vi "EIC_DIRC_DAQ_labview - kiethley.vi"() -> ()   [LabVIEW 2024]
uses:
  <instrlib>/Keithley 6517/Keithley 6517.lvlib
  O:/DSG/Tyler/EIC/DIRC/daq/automated/Thorlabs.MotionControl.Controls.dll
  Thorlabs.MotionControl.Controls.dll
  O:/DSG/Tyler/EIC/DIRC/daq/automated/Thorlabs.MotionControl.IntegratedStepperMotorsCLI.dll
  Thorlabs.MotionControl.IntegratedStepperMotorsCLI.dll
  O:/DSG/Tyler/EIC/DIRC/daq/automated/Thorlabs.MotionControl.DeviceManagerCLI.dll
  Thorlabs.MotionControl.DeviceManagerCLI.dll
panel:
  out "pdx_pos":dbl
  out "GetPositionCounter":i32
  out "pdy_dev":refnum<k24>
  out "pdx_dev":refnum<k24>
  in  "auto-align":bool
  out "meter-ref":string
  out "pd_rot_error":errorcluster
  out "brewster_rot_error":errorcluster
  in  "PD X":refnum<k24>(container)
  out "pd_rot_ref":refnum<k24>
  out "brewster_rot_ref":refnum<k24>
  in  "PD Angle":refnum<k24>(container)
  in  "Brewster":refnum<k24>(container)
  out "bary_error":errorcluster
  out "bary_ref":refnum<k24>
  out "barx_error":errorcluster
  out "barx_ref":refnum<k24>
  out "pdy_error":errorcluster
  out "pdy_ref":refnum<k24>
  out "pdx_error":errorcluster
  out "pdx_ref":refnum<k24>
  out "serial-numbers":string[](array[string])=["45000001", "45000002", "45000003", "45000004"]
  out "sim-instance":refnum<k24>
  in  "BAR Y":refnum<k24>(container)
  in  "BAR X":refnum<k24>(container)
  in  "PD Y":refnum<k24>(container)
  in  "dev-mode":bool
  out "start-msg":string
  in  "nSamples":dbl=50.0 caption="# Samples"
  in  "bar-note":bool
  out "sensor-stat":bool caption="Log Status"
  out "fout-stat":bool caption="Log Status"
  out "last-save":string caption="Last Save:"
  in  "save-data":bool
  out "Current Time:":string
  out "file-error":errorcluster
  out "log-path":path caption="Data will be saved at:"
  out "meter-error":errorcluster
  out "pd1_v":dbl caption="PD 1" format="%#.4g"
  out "pd2_v":dbl caption="PD 2" format="%#.4g"
  out "pd3_v":dbl caption="PD 3" format="%#.4g"
  out "pd-plt":cluster{"[0]":dbl, "[1]":dbl, "[2]":dbl}(graph) caption="Measurement History"
  in  "stop":bool
  # "PRESS STOP BEFORE \nCLOSING WINDOW"
  # "A"
  # "A"
  # "A"
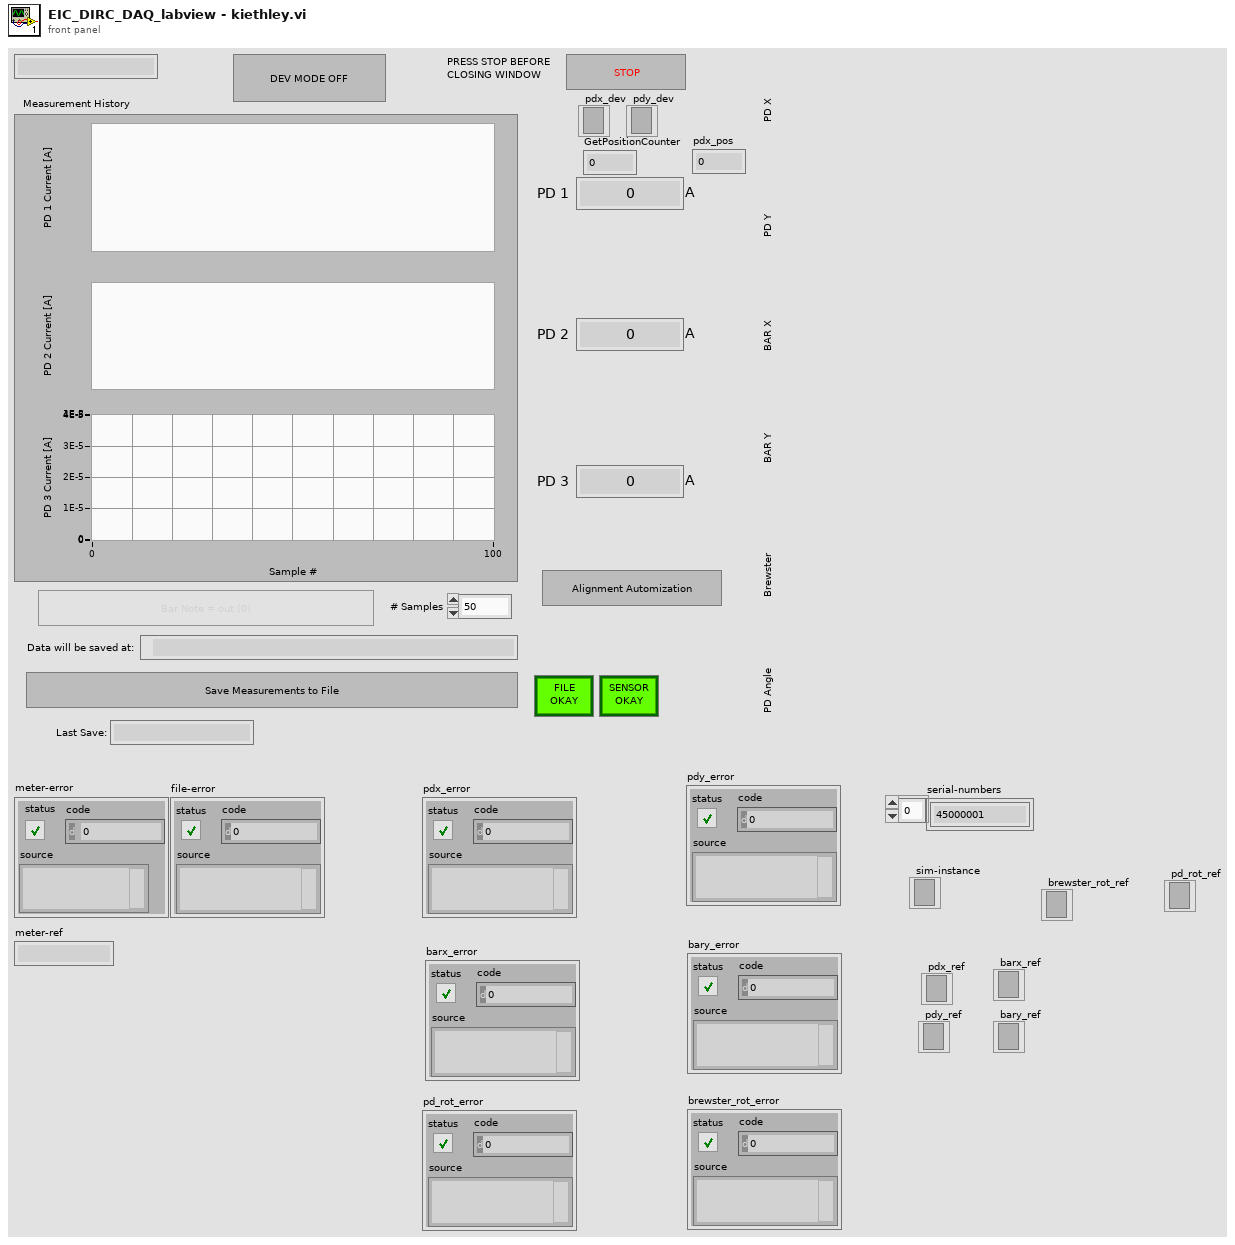
[diagram p1: front panel]
types:
  T1 = enum16{"PD X", "PD Y", "Bar X", "Bar Y", "Rotary"}
  T2 = enum16{"open", "replace", "create", "open or create", "replace or create", "replace or create with confirmation"}
  T3 = cluster{"error":bool, "code":i32, "source":string}
  T4 = cluster{"measurement":dbl, "measurement":dbl, "measurement":dbl}
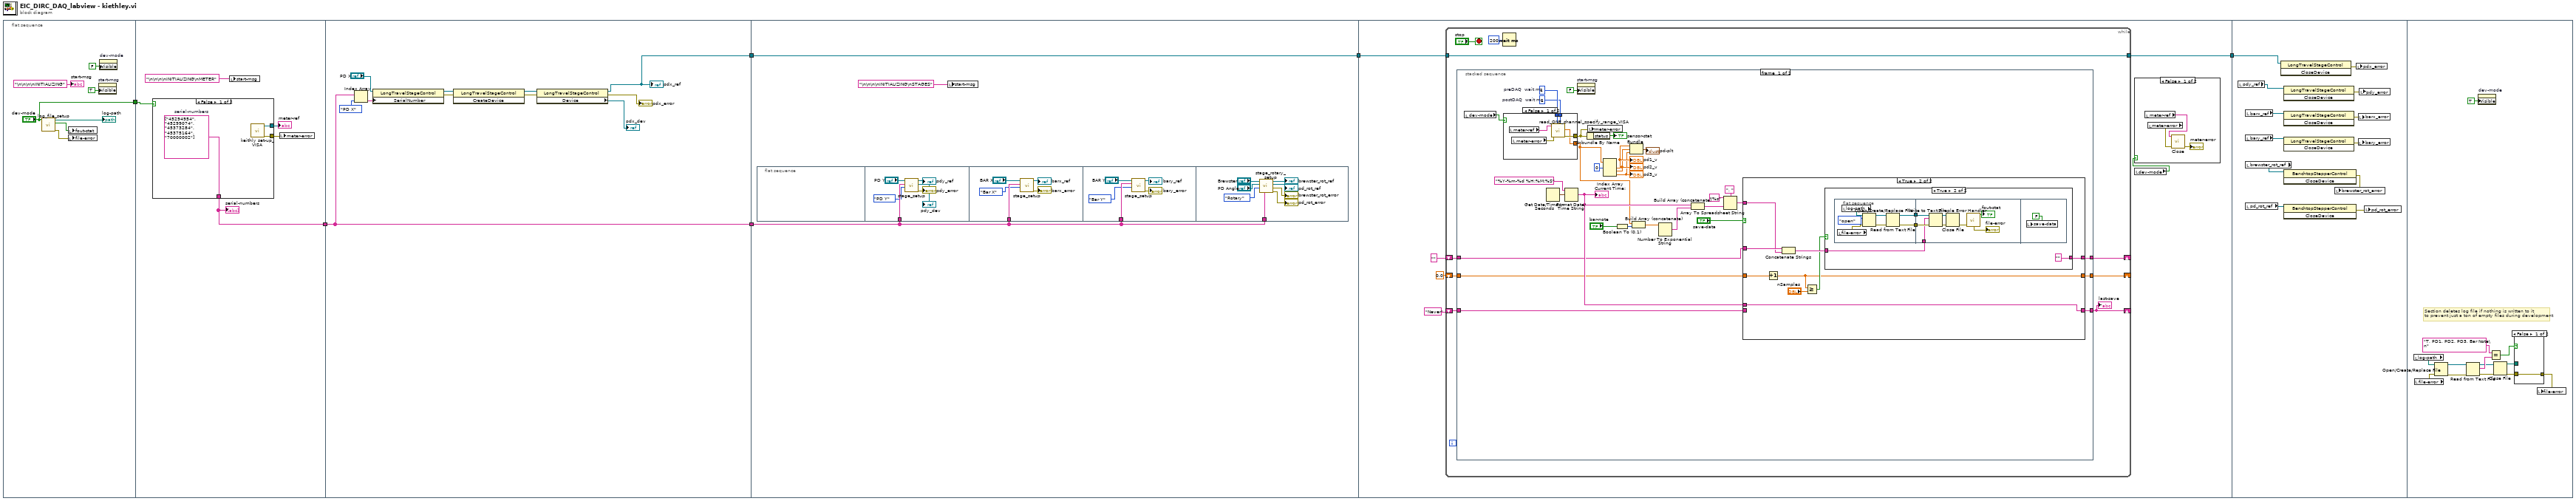
[diagram p0: block diagram]
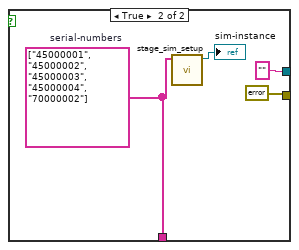
[diagram p2: hidden frame]
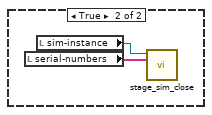
[diagram p3: hidden frame]
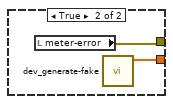
[diagram p4: hidden frame]
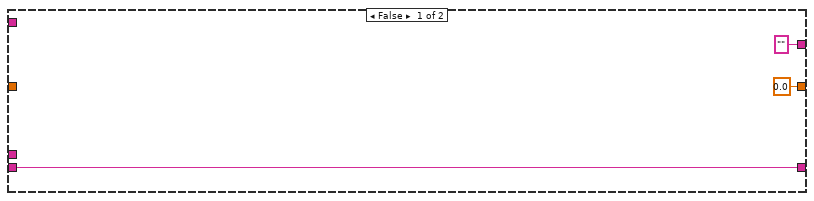
[diagram p5: hidden frame]
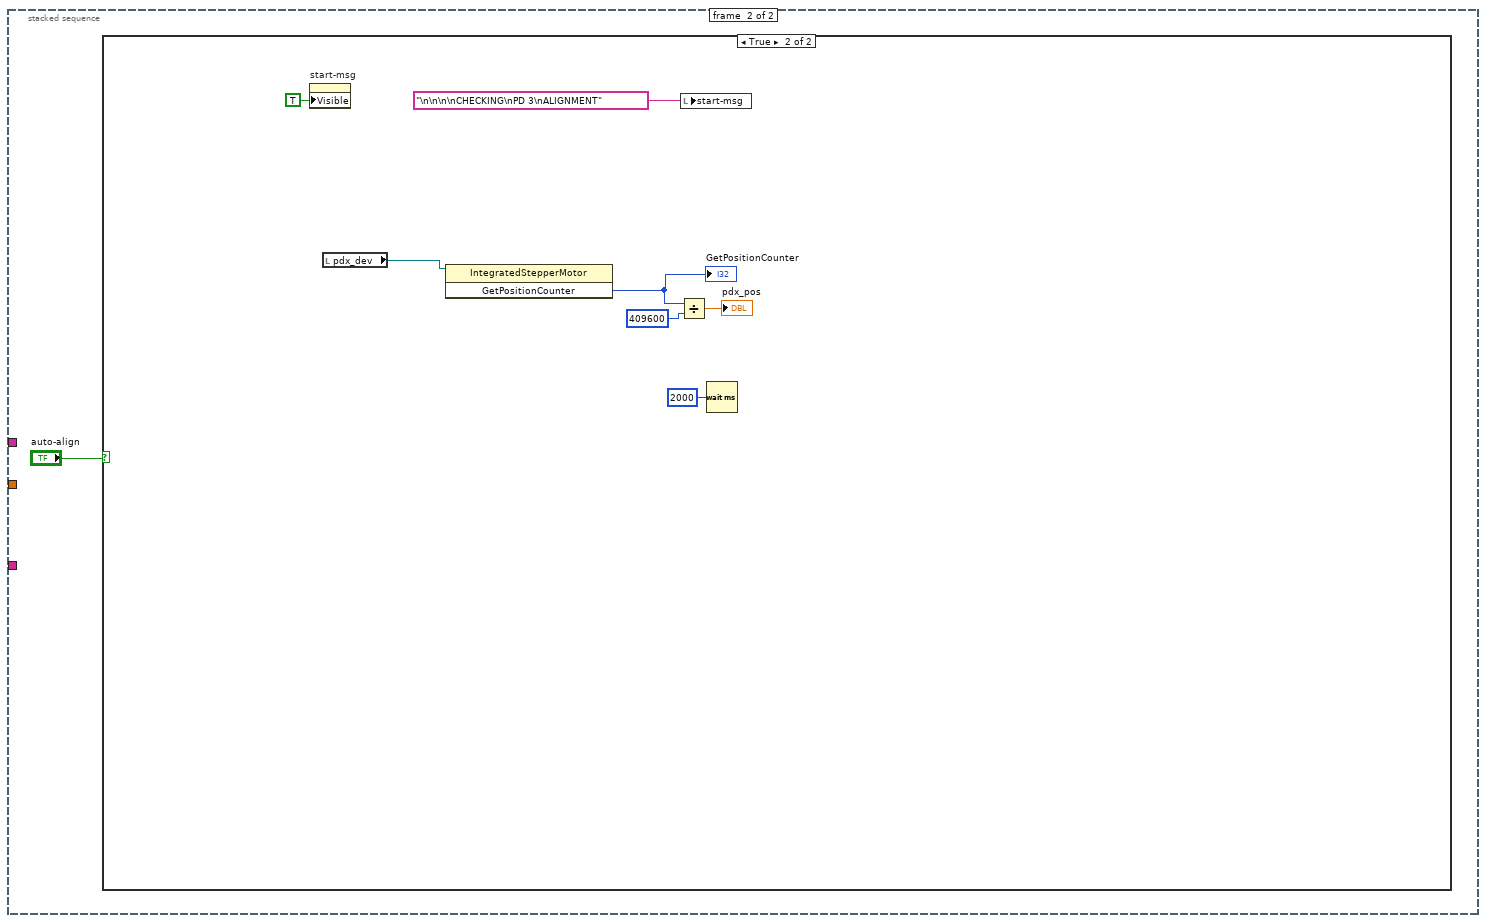
[diagram p7: hidden frame]
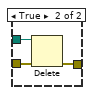
[diagram p9: hidden frame]
diagram:
  n1 = flat-sequence {
    tunnel: ["dev-mode"] -> w6
    tunnel: w6 -> [w17]
    tunnel: [w16] -> w3
    tunnel: w3 -> [w30]
    tunnel: [w30] -> w2
    tunnel: [w28] -> w1
    tunnel: w2 -> [w39]
    tunnel: [w37] -> w5
    tunnel: w1 -> [w37]
    tunnel: w5 -> [w65]
    tunnel: [w64] -> w4
    tunnel: w4 -> [w164]
    frame #0 {
      n2 = call "log_file_setup.vi"("dev-mode"="dev-mode") -> ("error out"=w11:errorcluster, "error?"=w12:bool, "appended path"=→"log-path":path)  [unwired: 8 in]
      n3 = local write "fout-stat"(w12) -> ()
      n4 = local write "file-error"(w11) -> ()
      n5 = property on="start-msg" class="Str"("Visible"=TRUE) -> ()  [unwired: 2 in, 2 out]
      n6 = property on="dev-mode" class="Bool (strict)"("Visible"=FALSE) -> ()  [unwired: 2 in, 2 out]
      "start-msg" <- "\n\n\n\nINITIALIZING" ("String")
    }
    frame #1 {
      n7 = case shown="False" w17 {
        tunnel: [w21 errorcluster {"status"=FALSE, "code"=0, "source"=""} ("error out")] -> w14
        tunnel: [w20 "" ("GPIB Address out")] -> w18
        tunnel: [w19 w22] -> w16
        frame False {
          w19 = string[] ["45294954", "45299074", "45373284", "45375164", "70000002"]  # serial-numbers
          n8 = call "keithly set-up_VISA.vi"() -> ("error out"=w21:errorcluster, "meter-VISA"=w20:refnum<visa-resource-name>)  [unwired: 10 in]
        }
        frame True {
          w22 = string[] ["45000001", "45000002", "45000003", "45000004", "70000002"]  # serial-numbers
          n9 = call "stage_sim_setup.vi"("serial-numbers"=w22) -> (".NET Refnum out"=→"sim-instance":refnum<k24>)  [unwired: 10 in]
        }
      }
      "serial-numbers" <- w16
      "meter-ref" <- w18
      n10 = local write "start-msg"("\n\n\n\nINITIALIZING\nMETER" ("String")) -> ()
      n11 = local write "meter-error"(w14) -> ()
    }
    frame #2 {
      n12 = Index Array(array=w30, index=T1."PD X" ("stage-select")) -> (element=w35:string)
      n13 = property class="LongTravelStageControl"(reference="PD X", "SerialNumber"=w35) -> (reference out=w34:refnum<k24>, error out=w33:errorcluster)  [unwired: 1 in]
      n14 = invoke class="LongTravelStageControl" method="CreateDevice"(reference=w34, error in=w33) -> (reference out=w32:refnum<k24>, error out=w31:errorcluster)  [unwired: 1 in, 1 out]
      n15 = property class="LongTravelStageControl"(reference=w32, error in=w31) -> (reference out=w28:refnum<k24>, error out=→"pdx_error":errorcluster, "Device"=→"pdx_dev":refnum<k24>)
      "pdx_ref" <- w28
    }
    frame #3 {
      n16 = flat-sequence {
        tunnel: w39 -> [w43]
        tunnel: w39 -> [w47]
        tunnel: w39 -> [w52]
        tunnel: w39 -> [w63]
        frame #0 {
        }
        frame #1 {
          n17 = call "stage_setup.vi"("stage-select"=enum16{"PD X", "PD Y", "Bar X", "Bar Y"}."PD Y", "serial-numbers"=w43, ".NET Refnum in"="PD Y") -> ("error out"=→"pdy_error":errorcluster, "Device"=→"pdy_dev":refnum<k24>, ".NET Refnum out"=→"pdy_ref":refnum<k24>)  [unwired: 6 in]
        }
        frame #2 {
          n18 = call "stage_setup.vi"("stage-select"=enum16{"PD X", "PD Y", "Bar X", "Bar Y"}."Bar X", "serial-numbers"=w47, ".NET Refnum in"="BAR X") -> ("error out"=→"barx_error":errorcluster, ".NET Refnum out"=→"barx_ref":refnum<k24>)  [unwired: 6 in, 1 out]
        }
        frame #3 {
          n19 = call "stage_setup.vi"("stage-select"=enum16{"PD X", "PD Y", "Bar X", "Bar Y"}."Bar Y", "serial-numbers"=w52, ".NET Refnum in"="BAR Y") -> ("error out"=→"bary_error":errorcluster, ".NET Refnum out"=→"bary_ref":refnum<k24>)  [unwired: 6 in, 1 out]
        }
        frame #4 {
          n20 = call "stage_rotary_setup.vi"("serial-numbers"=w63, "stage-select"=T1."Rotary", "ch2_ref_in"="PD Angle", "ch1_ref_in"="Brewster") -> ("ch2_error"=→"pd_rot_error":errorcluster, "ch1_error"=→"brewster_rot_error":errorcluster, "ch2_ref"=→"pd_rot_ref":refnum<k24>, "ch1_ref"=→"brewster_rot_ref":refnum<k24>)  [unwired: 2 in, 2 out]
        }
      }
      n21 = local write "start-msg"("\n\n\n\nINITIALIZING\nSTAGES" ("String")) -> ()
    }
    frame #4 {
      n22 = while {
        shift-right: [w80] -> _
        shift-left: "Never" -> [w81]
        shift-right: [w79] -> _
        shift-left: "" -> [w76]
        shift-right: [w77] -> _
        shift-left: 0.0 -> [w78]
        tunnel: w65 -> [w75]
        tunnel: [w75] -> w64
        stop <- "stop" stop-if-true
        n23 = stacked-sequence {
          tunnel: w81 -> [w104 _]
          tunnel: [w103 _] -> w80
          tunnel: [w89 _] -> w79
          tunnel: w78 -> [w88 _]
          tunnel: [w87 _] -> w77
          tunnel: w76 -> [w85 _]
          frame #0 {
            w94 = u32 1  # postDAQ  wait ms
            w95 = u32 1  # preDAQ  wait ms
            n24 = local read "dev-mode"() -> (w86:bool)
            n25 = case shown="False" w86 {
              tunnel: [w119 w120] -> w100
              tunnel: w95 -> [w118 _]
              tunnel: w94 -> [w117 _]
              tunnel: [w116 w121] -> w91
              frame False {
                n26 = local read "meter-ref"() -> (w114:string)
                n27 = local read "meter-error"() -> (w115:errorcluster)
                n28 = call "read_ONE_channel_specify_range_VISA.vi"("postDAQ  wait ms"=w117, "preDAQ  wait ms"=w118, "error in"=w115, "VISA resource in"=w114) -> ("error out"=w119:T3, "data"=w116:dbl[])  [unwired: 5 in, 1 out]
              }
              frame True {
                n29 = local read "meter-error"() -> (w120:errorcluster)
                n30 = call "dev_generate-fake.vi"() -> ("Array"=w121:dbl[])  [unwired: 11 in]
              }
            }
            n31 = Get Date/Time In Seconds() -> (seconds since 1Jan1904=w111:timestamp)
            n32 = Format Date/Time String(time format string (%c)="%Y-%m-%d %H:%M:%S", seconds (now)=w111) -> (date/time string=w105:string)  [unwired: 1 in]
            "Current Time:" <- w105
            n33 = property on="start-msg" class="Str"("Visible"=FALSE) -> ()  [unwired: 2 in, 2 out]
            n34 = Unbundle By Name(w100) -> ("status"=→"sensor-stat":bool)
            n35 = local write "meter-error"(w100) -> ()
            n36 = Index Array(array=w91, index #1=0 ("index")) -> (element #1=w99:dbl, element #2=w98:dbl, element #3=w97:dbl)  [unwired: 2 in]
            "pd3_v" <- w97
            "pd2_v" <- w98
            "pd1_v" <- w99
            n37 = Boolean To (0,1)(Boolean="bar-note") -> (0, 1=w90:i16)
            n38 = Bundle("measurement"=w99, "measurement"=w98, "measurement"=w97) -> (→"pd-plt":T4)  [unwired: 1 in]
            n39 = Build Array (concatenate)(w91, w90) -> (w92:dbl[])
            n40 = Number To Exponential String(number=w92) -> (E-format string=w96:string[])  [unwired: 3 in]
            n41 = Build Array (concatenate)(w105, w96) -> (w109:string[])
            n42 = Array To Spreadsheet String(delimiter (Tab)=", ", array=w109, 3:"%s" ("format string")) -> (spreadsheet string=w102:string)
            n43 = case shown="True" "save-data" {
              tunnel: w105 -> [_ w133]
              tunnel: [w124 w133] -> w103
              tunnel: w104 -> [w124 _]
              tunnel: w102 -> [_ w131]
              tunnel: w85 -> [_ w132]
              tunnel: ["" w129] -> w89
              tunnel: w88 -> [_ w128]
              tunnel: [0.0 w125] -> w87
              frame False {
              }
              frame True {
                n44 = Increment(x=w128) -> (x+1=w125:dbl)
                n45 = Concatenate Strings(w132, w131) -> (w130:string)
                n46 = Greater Or Equal?(x=w125, y="nSamples") -> (x >= y?=w126:bool)
                n47 = case shown="True" w126 {
                  tunnel: w130 -> [w134 w136]
                  tunnel: [w134 ""] -> w129
                  frame False {
                  }
                  frame True {
                    n48 = flat-sequence {
                      tunnel: [w141] -> w138
                      tunnel: [w143] -> w137
                      tunnel: w138 -> [w152]
                      tunnel: w137 -> [w151]
                      tunnel: w136 -> [w146]
                      frame #0 {
                        n49 = local read "file-error"() -> (w139:errorcluster)
                        n50 = local read "log-path"() -> (w140:path)
                        n51 = Open/Create/Replace File(file path (use dialog)=w140, error in=w139, operation (0:open)=T2."open") -> (refnum out=w144:refnum<file>, error out=w142:errorcluster)  [unwired: 3 in, 1 out]
                        n52 = Read from Text File(file (use dialog)=w144, error in=w142) -> (refnum out=w143:refnum<file>, error out=w141:errorcluster)  [unwired: 2 in, 2 out]
                      }
                      frame #1 {
                        n53 = Write to Text File(file (use dialog)=w151, text=w146, error in=w152) -> (refnum out=w150:refnum<file>, error out=w153:errorcluster)  [unwired: 1 in, 1 out]
                        n54 = Close File(refnum=w150, error in=w153) -> (error out=w149:errorcluster)  [unwired: 1 out]
                        n55 = call <vilib>:"Simple Error Handler.vi"("error in (no error)"=w149) -> ("error?"=→"fout-stat":bool, "error out"=→"file-error":errorcluster)  [unwired: 4 in, 3 out]
                      }
                      frame #2 {
                        n56 = local write "save-data"(FALSE ("save-data")) -> ()
                      }
                    }
                  }
                }
              }
            }
          }
          frame #1 {
            n57 = case shown="True" "auto-align" {
              frame False {
              }
              frame True {
                n58 = property on="start-msg" class="Str"("Visible"=TRUE) -> ()  [unwired: 2 in, 2 out]
                n59 = local read "pdx_dev"() -> (w159:refnum<k24>)
                n60 = invoke class="IntegratedStepperMotor" method="GetPositionCounter"(reference=w159) -> ("GetPositionCounter"=w158:i32)  [unwired: 2 in, 2 out]
                "GetPositionCounter" <- w158
                n61 = Divide(x=w158, y=409600 ("GetPositionCounter")) -> (x/y=→"pdx_pos":dbl)
                n62 = local write "start-msg"("\n\n\n\nCHECKING\nPD 3\nALIGNMENT" ("String")) -> ()
                n63 = Wait (ms)(milliseconds to wait=u32 2000) -> ()  [unwired: 1 out]
              }
            }
          }
        }
        "last-save" <- w80
        n64 = Wait (ms)(milliseconds to wait=u32 200) -> ()  [unwired: 1 out]
      }
      n65 = local read "dev-mode"() -> (w66:bool)
      n66 = case shown="False" w66 {
        frame False {
          n67 = local read "meter-ref"() -> (w70:string)
          n68 = local read "meter-error"() -> (w71:errorcluster)
          n69 = call <instrlib>:"Close.vi"("error in (no error)"=w71, "VISA resource name"=w70) -> ("error out"=→"meter-error":errorcluster)  [unwired: 9 in]
        }
        frame True {
          n70 = local read "serial-numbers"() -> (w74:string[])
          n71 = local read "sim-instance"() -> (w73:refnum<k24>)
          n72 = call "stage_sim_close.vi"("serial-numbers"=w74, ".NET Refnum in"=w73) -> ()  [unwired: 10 in]
        }
      }
    }
    frame #5 {
      n73 = local read "pdy_ref"() -> (w163:refnum<k24>)
      n74 = local read "barx_ref"() -> (w172:refnum<k24>)
      n75 = local read "bary_ref"() -> (w169:refnum<k24>)
      n76 = local read "brewster_rot_ref"() -> (w168:refnum<k24>)
      n77 = local read "pd_rot_ref"() -> (w167:refnum<k24>)
      n78 = invoke class="LongTravelStageControl" method="CloseDevice"(reference=w164) -> (error out=w174:errorcluster)  [unwired: 2 in, 2 out]
      n79 = invoke class="LongTravelStageControl" method="CloseDevice"(reference=w163) -> (error out=w173:errorcluster)  [unwired: 2 in, 2 out]
      n80 = invoke class="LongTravelStageControl" method="CloseDevice"(reference=w172) -> (error out=w171:errorcluster)  [unwired: 2 in, 2 out]
      n81 = invoke class="LongTravelStageControl" method="CloseDevice"(reference=w169) -> (error out=w170:errorcluster)  [unwired: 2 in, 2 out]
      n82 = invoke class="BenchtopStepperControl" method="CloseDevice"(reference=w168) -> (error out=w165:errorcluster)  [unwired: 2 in, 2 out]
      n83 = invoke class="BenchtopStepperControl" method="CloseDevice"(reference=w167) -> (error out=w166:errorcluster)  [unwired: 2 in, 2 out]
      n84 = local write "brewster_rot_error"(w165) -> ()
      n85 = local write "pdx_error"(w174) -> ()
      n86 = local write "barx_error"(w171) -> ()
      n87 = local write "bary_error"(w170) -> ()
      n88 = local write "pdy_error"(w173) -> ()
      n89 = local write "pd_rot_error"(w166) -> ()
    }
    frame #6 {
      # "Section deletes log file if nothing is written to it\nto prevent just a ton of empty files during development"
      n90 = local read "log-path"() -> (w175:path)
      n91 = local read "file-error"() -> (w182:errorcluster)
      n92 = Open/Create/Replace File(file path (use dialog)=w175, error in=w182) -> (refnum out=w187:refnum<file>, error out=w186:errorcluster)  [unwired: 4 in, 1 out]
      n93 = Read from Text File(file (use dialog)=w187, error in=w186) -> (refnum out=w184:refnum<file>, text=w185:string, error out=w183:errorcluster)  [unwired: 2 in, 1 out]
      n94 = property on="dev-mode" class="Bool (strict)"("Visible"=TRUE) -> ()  [unwired: 2 in, 2 out]
      n95 = Equal?(x="T, PD1, PD2, PD3, Bar Note\n" ("Display"), y=w185) -> (x = y?=w181:bool)
      n96 = Close File(refnum=w184, error in=w183) -> (path=w180:path, error out=w179:errorcluster)
      n97 = case shown="False" w181 {
        tunnel: w180 -> [_ w191]
        tunnel: w179 -> [w188 w190]
        tunnel: [w188 w189] -> w178
        frame False {
        }
        frame True {
          n98 = Delete(path (use dialog)=w191, error in=w190) -> (error out=w189:errorcluster)  [unwired: 3 in, 2 out]
        }
      }
      n99 = local write "file-error"(w178) -> ()
    }
  }
